vi "medicaoIXV.vi"() -> ()   [LabVIEW 2012]
uses:
  <vilib>/Utility/file.llb/Write To Spreadsheet File (string).vi
  <vilib>/Utility/file.llb/Write To Spreadsheet File (DBL).vi
  <instrlib>/Agilent 6XXX Series/Agilent 6XXX Series.lvlib
panel:
  out "reset graph":bool=TRUE
  out "tabela":dbl[][](array[numeric])
  in  "Tab Control":enum32{"Entrada de dados", "Saída de dados"}(tab)
  in  "Área da célula":dbl
  in  "Tipo da célula":string
  in  "Formato":u16(ring) items=[".txt", ".csv"]
  out "ON/OFF1":bool caption="ON/OFF"
  in  "Pontos":dbl
  in  "Tensão máxima":dbl
  in  "Nome da célula":string
  in  "Local":path
  in  "Delay(ms)":dbl
  in  "Start":bool
  in  "stopProgram":bool caption="Parar Programa"
  out "Imp":dbl
  out "Vmp":dbl
  out "Pmp":dbl
  out "Icc (A)":dbl
  out "Vca (V)":dbl
  in  "Print Screen":bool
  out "IXV":cluster{"Y":dbl[], "Y":dbl[]}[](graph)
  out "output voltage":dbl
  out "Tensao Atual (V)":dbl
  out "Corrente Atual\n(A)":dbl
  out "Ponto Atual":i32
  out "tabela":dbl[][](array[numeric]) caption="TABELA DE DADOS\nTensão(Fonte)      Pontos             Tensao           Corrente" format="%0.3f"
  in  "stop":bool caption="Parar Medição"
  out "ON/OFF2":bool caption="ON/OFF"
  in  "CorrenteGraph":dbl
  in  "error in (no error)":errorcluster
  out "error out":errorcluster
  in  "TensaoGraph":dbl
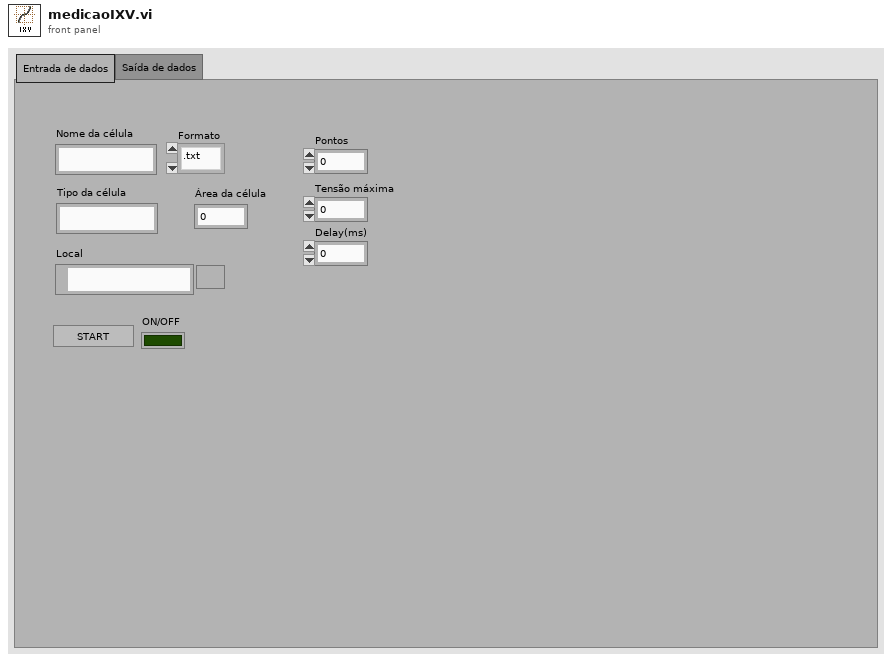
[diagram p1: front panel]
types:
  T1 = typedef "imagedata.ctl" = cluster{"image type":i32, "image depth":i32, "image":u8[], "mask":u8[], "colors":u32[], "Rectangle":cluster{"left":i16, "top":i16, "right":i16, "bottom":i16}}
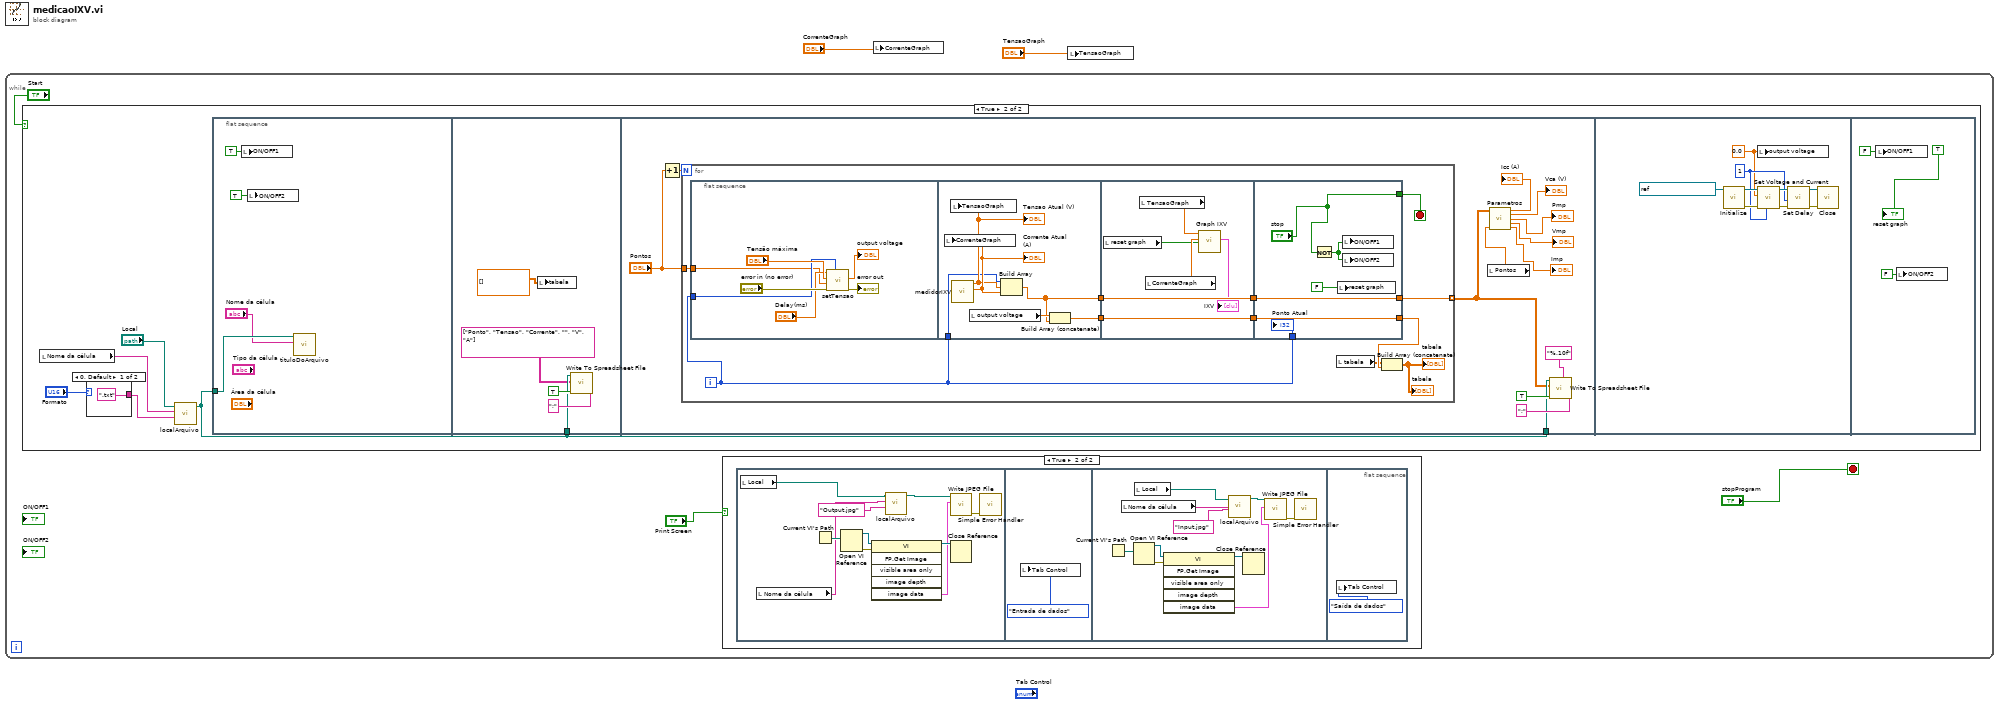
[diagram p0: block diagram]
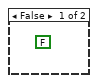
[diagram p3: hidden frame]
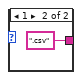
[diagram p4: hidden frame]
diagram:
  n1 = while {
    stop <- "stopProgram" stop-if-true
    n2 = case shown="True" "Start" {
      frame False {
        (unwired) FALSE
      }
      frame True {
        n3 = local read "Nome da célula"() -> (w31:string)
        n4 = case shown="0, Default" "Formato" {
          tunnel: [".txt" ".csv"] -> w28
          frame 0, Default {
          }
          frame 1 {
          }
        }
        n5 = call "localArquivo.vi"("extensão"=w28, "Nome do arquivo"=w31, "Local"="Local") -> ("Path"=w30:path)  [unwired: 8 in]
        n6 = flat-sequence {
          tunnel: w30 -> [w38]
          tunnel: w30 -> [w41]
          tunnel: w30 -> [w54]
          frame #0 {
            n7 = local write "ON/OFF1"(TRUE ("ON/OFF")) -> ()
            n8 = local write "ON/OFF2"(TRUE ("ON/OFF2")) -> ()
            n9 = call "tituloDoArquivo.vi"("Nome da célula"="Nome da célula", "file path (dialog if empty)"=w38) -> ()  [unwired: 10 in]
          }
          frame #1 {
            n10 = local write "tabela"(dbl[][] [] ("array")) -> ()
            n11 = call-poly <vilib>:"Write To Spreadsheet File.vi"("delimiter (\\t)"=";" ("delimiter (\\t)"), "append to file? (new file:F)"=TRUE, "2D data"=string[][] [["Ponto", "Tensao", "Corrente"], ["", "V", "A"]], "file path (dialog if empty)"=w41) -> ()  [unwired: 4 in, 1 out]
          }
          frame #2 {
            n12 = Increment(x="Pontos") -> (x+1=w53:dbl)
            n13 = for {
              N: w53 -> [_]
              tunnel: [w66] -> w51 mode=indexing
              tunnel: "Pontos" -> [w67]
              i -> [w60]
              stop <- w59 stop-if-true
              n14 = flat-sequence {
                tunnel: w67 -> [w70]
                tunnel: w60 -> [w71]
                tunnel: w60 -> [w75]
                tunnel: [w78] -> w65
                tunnel: [w80] -> w64
                tunnel: [w86] -> w58
                tunnel: [w85] -> w57
                tunnel: w64 -> [w85]
                tunnel: w65 -> [w86]
                tunnel: [w91] -> w63
                tunnel: [w92] -> w66
                tunnel: w58 -> [w92]
                tunnel: w57 -> [w91]
                tunnel: w60 -> [w90]
                tunnel: ["stop"] -> w59
                frame #0 {
                  n15 = call "setTensao.vi"("Ponto"=w71, "error in (no error)"="error in (no error)", "Pontos"=w70, "Tensão máxima"="Tensão máxima", "delay(ms)"="Delay(ms)") -> ("error out"=→"error out":errorcluster, "output voltage"=→"output voltage":dbl)  [unwired: 5 in]
                }
                frame #1 {
                  n16 = call "medidorIXV.vi"() -> ("Corrente Atual"=w77:dbl, "Tensao Atual"=w76:dbl)  [unwired: 10 in]
                  "Corrente Atual\n(A)" <- w77
                  "Tensao Atual (V)" <- w76
                  n17 = local write "CorrenteGraph"(w77) -> ()
                  n18 = local write "TensaoGraph"(w76) -> ()
                  n19 = local read "output voltage"() -> (w79:dbl)
                  n20 = Build Array(w75, w76, w77) -> (w78:dbl[])
                  n21 = Build Array (concatenate)(w79, w78) -> (w80:dbl[])
                }
                frame #2 {
                  n22 = local read "reset graph"() -> (w81:bool)
                  n23 = local read "TensaoGraph"() -> (w84:dbl)
                  n24 = local read "CorrenteGraph"() -> (w83:dbl)
                  n25 = call "Graph IXV"("Reset"=w81, "Y Input"=w83, "X Input"=w84) -> ("XY Graph"=→"IXV":cluster{"Y":dbl[], "Y":dbl[]}[])  [unwired: 2 in, 6 out]
                }
                frame #3 {
                  n26 = Not(x="stop") -> (.not. x?=w88:bool)
                  n27 = local write "reset graph"(FALSE) -> ()
                  n28 = local write "ON/OFF1"(w88) -> ()
                  n29 = local write "ON/OFF2"(w88) -> ()
                  "Ponto Atual" <- w90
                }
              }
              n30 = local read "tabela"() -> (w62:dbl[][])
              n31 = Build Array (concatenate)(w62, w63) -> (→"tabela" →"tabela":dbl[][])
            }
            n32 = local read "Pontos"() -> (w50:dbl)
            n33 = call "Parametros.vi"("VetorDeDados"=w51, "pontos"=w50) -> ("Icc"=→"Icc (A)":dbl, "Vca"=→"Vca (V)":dbl, "Pmp"=→"Pmp":dbl, "Vmp"=→"Vmp":dbl, "Imp"=→"Imp":dbl)  [unwired: 9 in]
            n34 = call-poly <vilib>:"Write To Spreadsheet File.vi"("delimiter (\\t)"=";" ("delimiter (\\t)"), "format (%.3f)"="%.10f", "append to file? (new file:F)"=TRUE, "2D data"=w51, "file path (dialog if empty)"=w54) -> ()  [unwired: 3 in, 1 out]
          }
          frame #3 {
            w93 = 0.0 ("voltage (0 V)")
            w96 = u8 1 ("channel (1)")
            n35 = call <instrlib>:"Initialize.vi"("VISA resource name"=refnum<visa-resource-name> "GPIB0::5::INSTR") -> ("error out"=w98:errorcluster, "VISA resource name out"=w97:refnum<visa-resource-name>)  [unwired: 9 in]
            n36 = local write "output voltage"(w93) -> ()
            n37 = call <instrlib>:"Set Voltage and Current.vi"("channel (1)"=w96, "error in (no error)"=w98, "voltage (0 V)"=w93, "VISA resource name"=w97) -> ("error out"=w99:errorcluster, "VISA resource name out"=w100:refnum<visa-resource-name>)  [unwired: 6 in]
            n38 = call <instrlib>:"Set Delay.vi"("error in (no error)"=w99, "channel (1)"=w96, "VISA resource name"=w100) -> ("error out"=w94:errorcluster, "VISA resource name out"=w95:refnum<visa-resource-name>)  [unwired: 7 in]
            n39 = call <instrlib>:"Close.vi"("error in (no error)"=w94, "VISA resource name"=w95) -> ()  [unwired: 9 in, 1 out]
          }
          frame #4 {
            n40 = local write "ON/OFF1"(FALSE) -> ()
            n41 = local write "ON/OFF2"(FALSE ("ON/OFF")) -> ()
            "reset graph" <- TRUE
          }
        }
      }
    }
    n42 = case shown="True" "Print Screen" {
      frame False {
      }
      frame True {
        n43 = flat-sequence {
          frame #0 {
            n44 = local read "Local"() -> (w7:path)
            n45 = local read "Nome da célula"() -> (w8:string)
            n46 = Current VI's Path() -> (path=w13:path)
            n47 = Open VI Reference(vi path=w13) -> (vi reference=w14:refnum<vi>, error out=w15:errorcluster)  [unwired: 5 in]
            n48 = invoke class="VI" method="FP.Get Image"(reference=w14, error in=w15) -> (reference out=w12:refnum<vi>, "image data"=w11:T1)  [unwired: 4 in, 4 out]
            n49 = call "localArquivo.vi"("extensão"="Output.jpg", "Nome do arquivo"=w8, "Local"=w7) -> ("Path"=w6:path)  [unwired: 8 in]
            n50 = call <vilib>:"Write JPEG File.vi"("image data"=w11, "path to JPEG file"=w6) -> ("error out"=w10:errorcluster)  [unwired: 8 in, 1 out]
            n51 = Close Reference(reference=w12) -> ()  [unwired: 1 in, 1 out]
            n52 = call <vilib>:"Simple Error Handler.vi"("error in (no error)"=w10) -> ()  [unwired: 4 in, 5 out]
          }
          frame #1 {
            n53 = local write "Tab Control"(enum32{"Entrada de dados", "Saída de dados"}."Entrada de dados" ("Tab Control")) -> ()
          }
          frame #2 {
            n54 = Current VI's Path() -> (path=w25:path)
            n55 = local read "Nome da célula"() -> (w19:string)
            n56 = Open VI Reference(vi path=w25) -> (vi reference=w24:refnum<vi>, error out=w23:errorcluster)  [unwired: 5 in]
            n57 = local read "Local"() -> (w18:path)
            n58 = invoke class="VI" method="FP.Get Image"(reference=w24, error in=w23) -> (reference out=w26:refnum<vi>, "image data"=w21:T1)  [unwired: 4 in, 4 out]
            n59 = call "localArquivo.vi"("extensão"="Input.jpg", "Nome do arquivo"=w19, "Local"=w18) -> ("Path"=w17:path)  [unwired: 8 in]
            n60 = Close Reference(reference=w26) -> ()  [unwired: 1 in, 1 out]
            n61 = call <vilib>:"Write JPEG File.vi"("image data"=w21, "path to JPEG file"=w17) -> ("error out"=w22:errorcluster)  [unwired: 8 in, 1 out]
            n62 = call <vilib>:"Simple Error Handler.vi"("error in (no error)"=w22) -> ()  [unwired: 4 in, 5 out]
          }
          frame #3 {
            n63 = local write "Tab Control"(enum32{"Entrada de dados", "Saída de dados"}."Saída de dados" ("Tab Control")) -> ()
          }
        }
      }
    }
  }
  n64 = local write "CorrenteGraph"("CorrenteGraph") -> ()
  n65 = local write "TensaoGraph"("TensaoGraph") -> ()
